vi "GetisciFilemeasures_settings_INPUT.vi"(0 "Numero Misure":dbl, 1 "Array ClusterCaratteristicheMisura IN":T1[](array[typedef]), 2 "banco":i32, 6 "Azione":string) -> (7 "Array ClusterCaratteristicheMisura OUT":T1[](array[typedef]))   [LabVIEW 2019]
uses:
  TypeDef/ClusterCaratteristicheMisura_INPUT.ctl
  <vilib>/Utility/file.llb/Read Delimited Spreadsheet (string).vi
panel:
  in  "Cluster Caratteriestiche Misura":T1
  out "Lettura file txt":string[][](array[string])
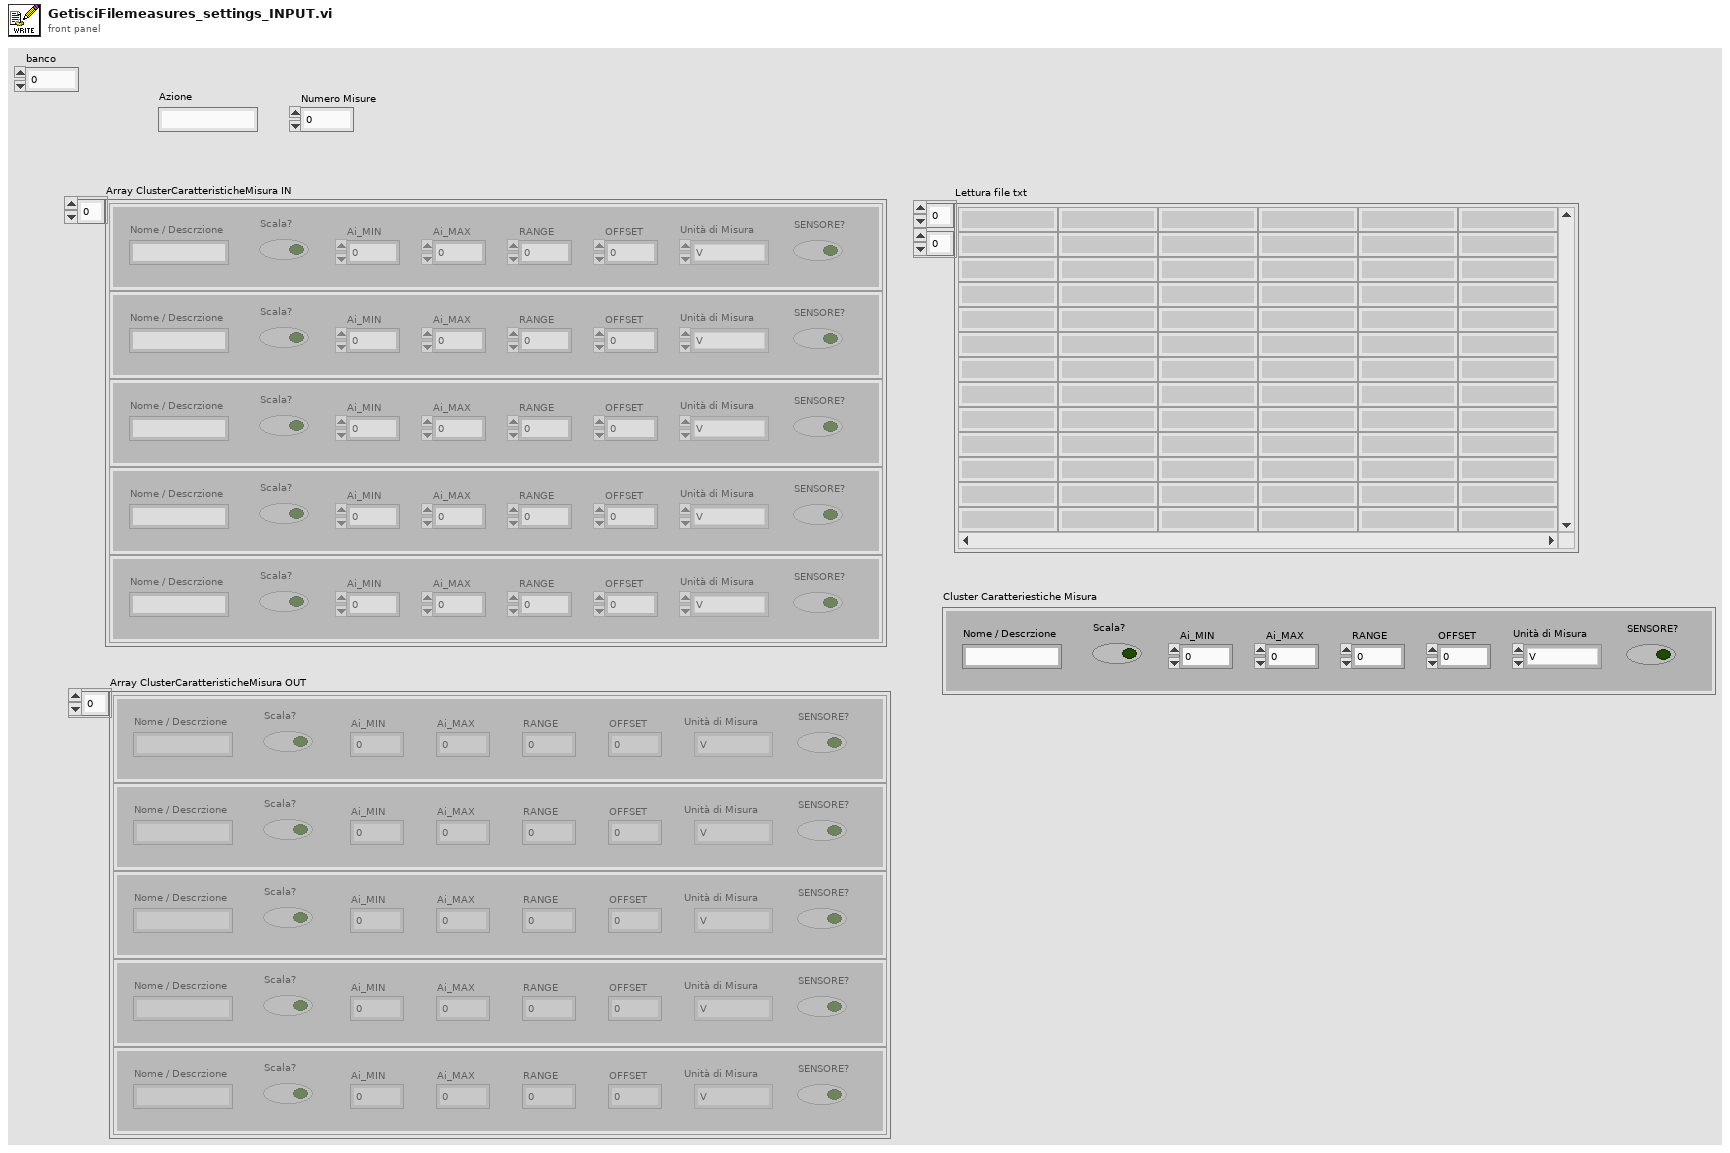
[diagram p1: front panel]
types:
  T1 = typedef "ClusterCaratteristicheMisura_INPUT.ctl" = cluster{"Nome / Descrzione":string, "Scala?":bool, "Ai_MIN":dbl, "Ai_MAX":dbl, "RANGE":dbl, "OFFSET":dbl, "Unità di Misura":T2, "SENSORE?":bool}
  T2 = typedef "UnitàMisura.ctl" = enum16{"V", "mA", "Bar", "RPM", "m3/s", "m3/min", "m3/h", "l/s", "l/min", "in3/min", "ft3/min", "gpm", "igpm", "igph", "%", "°C", "m", "Nm", "A"}
  T3 = enum16{"open", "replace", "create", "open or create", "replace or create", "replace or create with confirmation"}
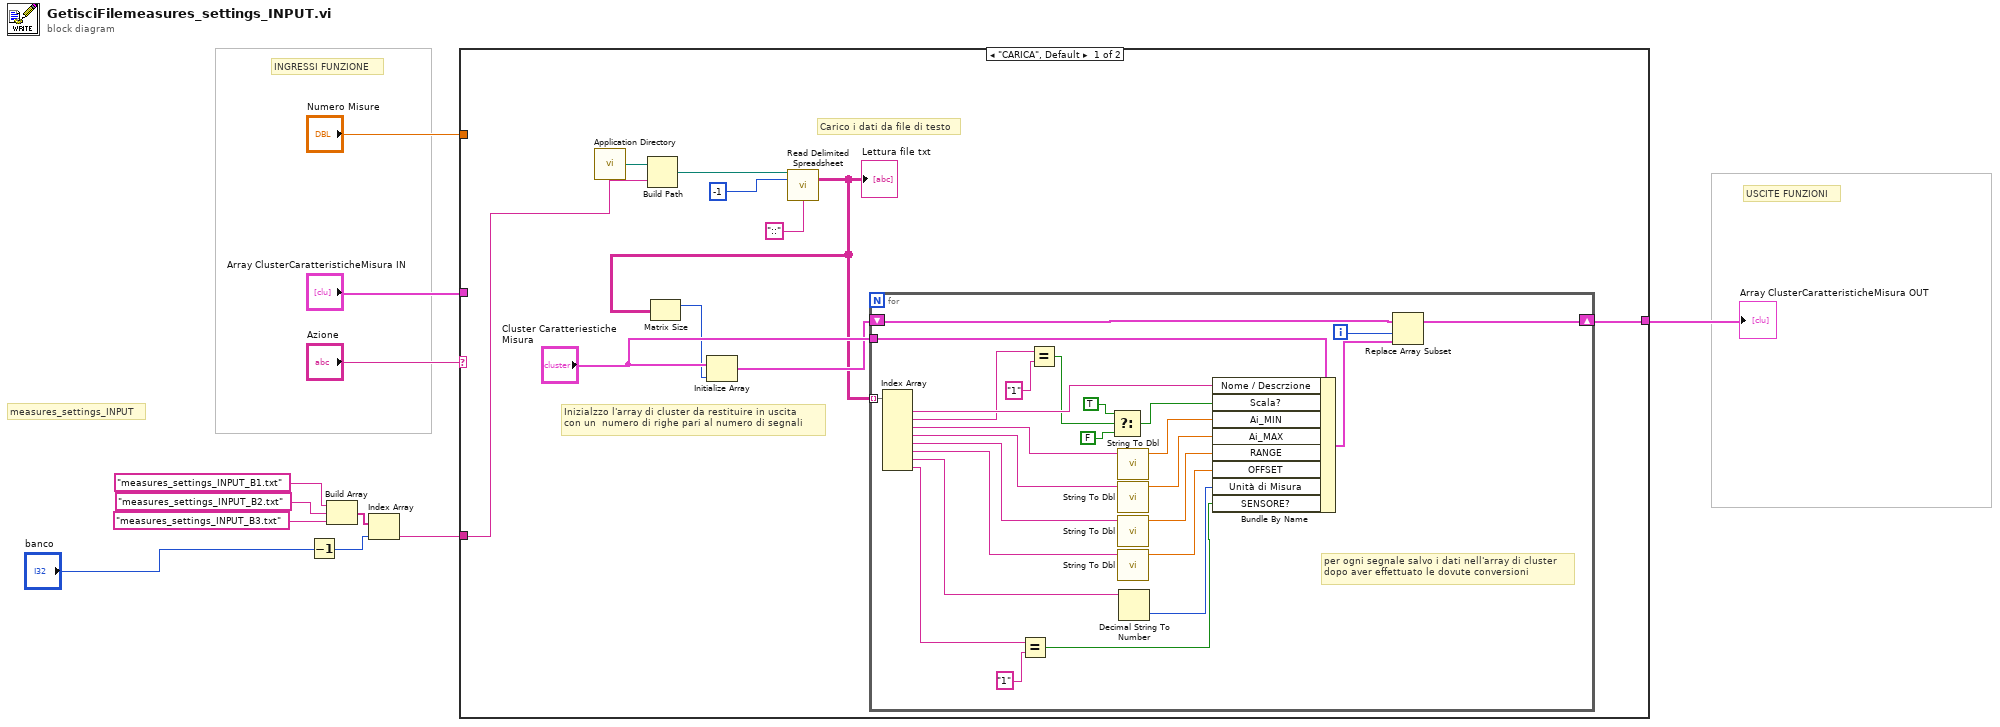
[diagram p0: block diagram]
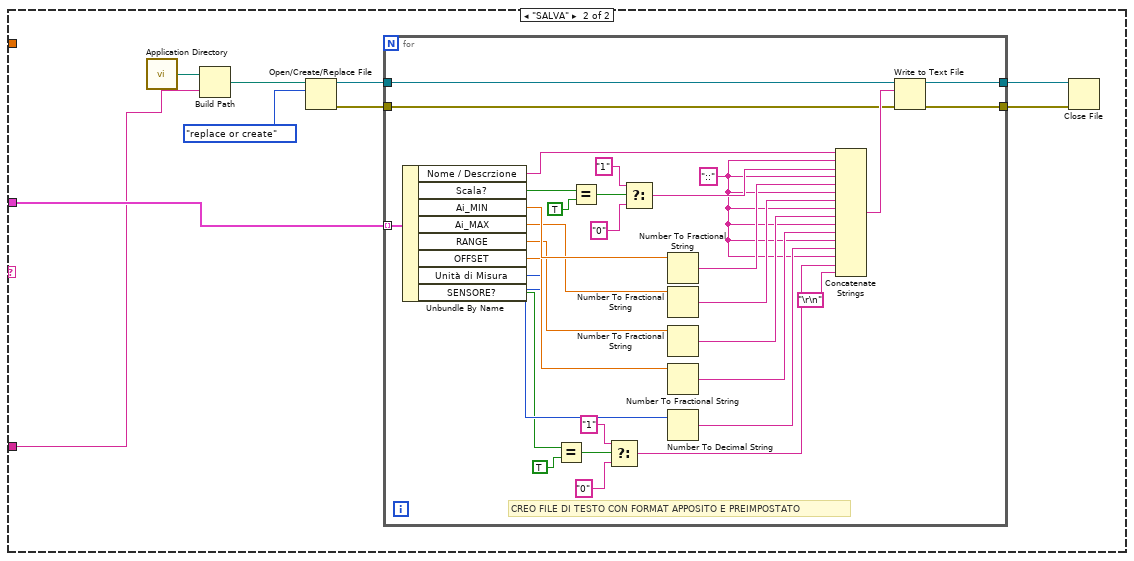
[diagram p2: hidden frame]
diagram:
  # "measures_settings_INPUT"
  # "USCITE FUNZIONI"
  # "INGRESSI FUNZIONE"
  n1 = Decrement(x="banco") -> (x-1=w3:i32)
  n2 = Build Array("measures_settings_INPUT_B1.txt" ("name or relative path"), "measures_settings_INPUT_B2.txt" ("name or relative path"), "measures_settings_INPUT_B3.txt" ("name or relative path")) -> (w4:string[])
  n3 = Index Array(array=w4, index=w3) -> (element=w1:string)
  n4 = case shown="\"CARICA\", Default" "Azione" {
    tunnel: "Array ClusterCaratteristicheMisura IN" -> [_ w49]
    tunnel: "Numero Misure" -> [_ _]
    tunnel: [w15 _] -> w8
    tunnel: w1 -> [w12 w48]
    frame "CARICA", Default {
      # "Inizialzzo l'array di cluster da restituire in uscita\ncon un  numero di righe pari al numero di segnali"
      # "Carico i dati da file di testo"
      n5 = call <vilib>:"Application Directory.vi"() -> ("Application Directory"=w21:path)
      n6 = Build Path(base path=w21, name or relative path=w12) -> (appended path=w20:path)
      n7 = call-poly <vilib>:"Read Delimited Spreadsheet.vi"("file path (dialog if empty)"=w20, "number of rows (all:-1)"=-1, "delimiter (\\t)"="::" ("delimiter (\\t)")) -> ("all rows"=w14:string[][])  [unwired: 7 in, 5 out]
      "Lettura file txt" <- w14
      n8 = Matrix Size(0:w14) -> (1:w13:i32)  [unwired: 1 out]
      n9 = Initialize Array("Cluster Caratteriestiche Misura", w13) -> (w16:T1[])
      n10 = for {
        tunnel: w14 -> [w47] mode=indexing
        tunnel: "Cluster Caratteriestiche Misura" -> [w37]
        shift-right: [w33] -> w15
        shift-left: w16 -> [w36]
        i -> [w34]
        # "per ogni segnale salvo i dati nell'array di cluster \ndopo aver effettuato le dovute conversioni"
        n11 = Index Array(array=w47) -> (element #1=w46:string, element #2=w45:string, element #3=w29:string, element #4=w27:string, element #5=w26:string, element #6=w25:string, element #7=w39:string, element #8=w31:string)  [unwired: 8 in]
        n12 = Equal?(x=w31, y="1") -> (x = y?=w30:bool)
        n13 = Equal?(x=w45, y="1") -> (x = y?=w43:bool)
        n14 = Select(t=TRUE, s=w43, f=FALSE) -> (s? t:f=w40:bool)
        n15 = call "String To Dbl.vi"("String"=w29) -> ("Numeric"=w28:dbl)  [unwired: 10 in]
        n16 = call "String To Dbl.vi"("String"=w27) -> ("Numeric"=w24:dbl)  [unwired: 10 in]
        n17 = call "String To Dbl.vi"("String"=w26) -> ("Numeric"=w23:dbl)  [unwired: 10 in]
        n18 = call "String To Dbl.vi"("String"=w25) -> ("Numeric"=w22:dbl)  [unwired: 10 in]
        n19 = Decimal String To Number(string=w39) -> (number=w38:i32)  [unwired: 2 in, 1 out]
        n20 = Bundle By Name(cluster=w37, "Nome / Descrzione"=w46, "Scala?"=w40, "Ai_MIN"=w28, "Ai_MAX"=w24, "RANGE"=w23, "OFFSET"=w22, "Unità di Misura"=w38, "SENSORE?"=w30) -> (w35:T1)
        n21 = Replace Array Subset(array=w36, new element=w35, index=w34) -> (w33:T1[])
      }
    }
    frame "SALVA" {
      n22 = call <vilib>:"Application Directory.vi"() -> ("Application Directory"=w56:path)
      n23 = Build Path(base path=w56, name or relative path=w48) -> (appended path=w54:path)
      n24 = Open/Create/Replace File(file path (use dialog)=w54, operation (0:open)=T3."replace or create") -> (refnum out=w55:refnum<file>, error out=w51:errorcluster)  [unwired: 4 in, 1 out]
      n25 = for {
        tunnel: w55 -> [w86]
        tunnel: w49 -> [w87] mode=indexing
        tunnel: [w73] -> w52
        tunnel: w51 -> [w72]
        tunnel: [w71] -> w50
        w58 = "::" ("string")
        # "CREO FILE DI TESTO CON FORMAT APPOSITO E PREIMPOSTATO"
        n26 = Unbundle By Name(w87) -> ("Nome / Descrzione"=w80:string, "Scala?"=w85:bool, "Ai_MIN"=w79:dbl, "Ai_MAX"=w78:dbl, "RANGE"=w77:dbl, "OFFSET"=w76:dbl, "Unità di Misura"=w75:T2, "SENSORE?"=w60:bool)
        n27 = Equal?(x=w60, y=TRUE) -> (x = y?=w64:bool)
        n28 = Equal?(x=w85, y=TRUE) -> (x = y?=w83:bool)
        n29 = Select(t="1", s=w64, f="0") -> (s? t:f=w59:string)
        n30 = Select(t="1", s=w83, f="0") -> (s? t:f=w70:string)
        n31 = Number To Fractional String(number=w79) -> (F-format string=w69:string)  [unwired: 3 in]
        n32 = Number To Fractional String(number=w78) -> (F-format string=w68:string)  [unwired: 3 in]
        n33 = Number To Fractional String(number=w77) -> (F-format string=w67:string)  [unwired: 3 in]
        n34 = Number To Fractional String(number=w76) -> (F-format string=w66:string)  [unwired: 3 in]
        n35 = Number To Decimal String(number=w75) -> (decimal integer string=w65:string)  [unwired: 1 in]
        n36 = Concatenate Strings(w80, w58, w70, w58, w69, w58, w68, w58, w67, w58, w66, w58, w65, w58, w59, "\r\n") -> (w74:string)
        n37 = Write to Text File(file (use dialog)=w86, text=w74, error in=w72) -> (refnum out=w73:refnum<file>, error out=w71:errorcluster)  [unwired: 1 in, 1 out]
      }
      n38 = Close File(refnum=w52, error in=w50) -> ()  [unwired: 2 out]
    }
  }
  "Array ClusterCaratteristicheMisura OUT" <- w8
